vi "acquireValue.vi"(8 "error in (no error)":errorcluster, 10 "nextSample?":bool, 11 "setMode in":refnum<class "setMode.lvclass">) -> (0 "error out":errorcluster, 1 "function return":i32, 2 "variantData":variant, 3 "setMode out":refnum<class "setMode.lvclass">)   [LabVIEW 2016, in "SALLV_MtAtElectrometer_Messaging.lvlib" / "setMode.lvclass"]
uses:
  setMode.lvclass
  ts_sallv_MtAtElectrometer/SALLV_MtAtElectrometer.lvlib
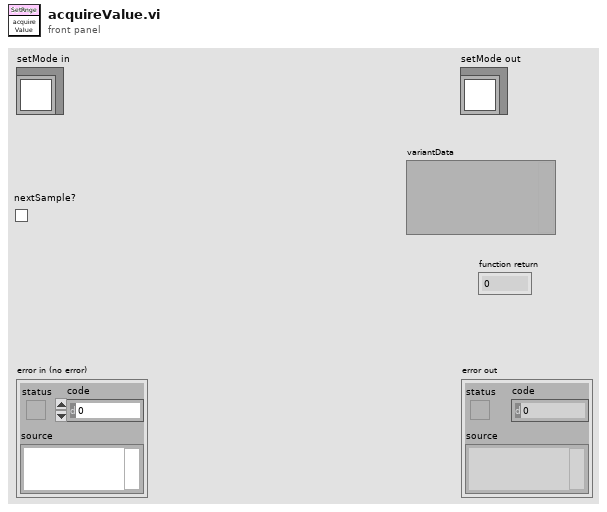
[diagram p1: front panel]
types:
  T1 = typedef "SALLV_MtAtElectrometer.lvlib/command_setMode.ctl" = cluster{"mode":u16}
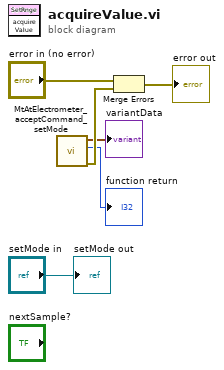
[diagram p0: block diagram]
diagram:
  n1 = call "MtAtElectrometer_acceptCommand_setMode.vi"() -> ("error out"=w3:errorcluster, "function return"=→"function return":i32, "command_setMode_Ctl out"=→"variantData":T1)  [unwired: 9 in]
  n2 = Merge Errors("error in (no error)", w3) -> (→"error out":errorcluster)
  "setMode out" <- "setMode in"
